vi "close_service.vi"(8 "error in (no error)":errorcluster, 11 "system.logging (in)":refnum<class "system.logging.lvclass">) -> (0 "error out":errorcluster, 3 "system.logging (out)":refnum<class "system.logging.lvclass">)   [LabVIEW 2021, in "system.logging.lvclass"]
uses:
  system.logging.lvclass
  system.logging.lvclass/system.logging.ctl
  service_commands.ctl
  severity.ctl
  log_entry.ctl
  log_stream.ctl
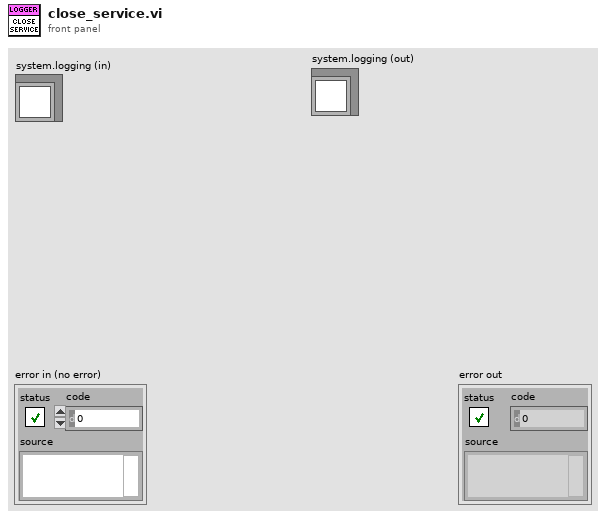
[diagram p1: front panel]
types:
  T1 = typedef "system.logging.lvclass/log_stream.ctl" = cluster{"command":T2, "log_entry":T3}
  T2 = typedef "system.logging.lvclass/service_commands.ctl" = enum16{"close", "log"}
  T3 = typedef "system.logging.lvclass/log_entry.ctl" = cluster{"severity":T4, "message":string, "origin":string, "datetime":timestamp}
  T4 = typedef "system.logging.lvclass/severity.ctl" = enum8{"trace", "debug", "info", "warning", "error"}
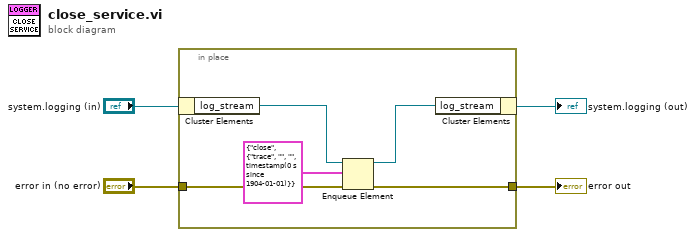
[diagram p0: block diagram]
diagram:
  n1 = in-place {
    in-place-border: "error in (no error)" -> [w9]
    in-place-border: [w6] -> w1
    n2 = in-place-cluster #1("system.logging (in)") -> ("log_stream"=w8:refnum<queue>)
    n3 = Enqueue Element(queue=w8, element=T1 {"command"=enum."close", "log_entry"={"severity"=enum."trace", "message"="", "origin"="", "datetime"=timestamp(0 s since 1904-01-01)}}, error in (no error)=w9) -> (queue out=w7:refnum<queue>, error out=w6:errorcluster)  [unwired: 1 in, 1 out]
    n4 = in-place-cluster #1("log_stream"=w7) -> (→"system.logging (out)":refnum<class "system.logging.lvclass">)
  }
  "error out" <- w1
